vi "Measurement Logic.vi"() -> ()   [LabVIEW 2021, in "niScope EX Getting Started.lvlib"]
uses:
  niScope EX Getting Started.lvlib
  Measurement Configuration.ctl
  Measurement Results.ctl
  <vilib>/Plug-In SDKs/Measurements/Measure Call Context/Measure Call Context.lvclass
  <vilib>/Plug-In SDKs/Sessions/niScope/NI Session Management niScope.lvlib
  <vilib>/Plug-In SDKs/Clients/Session Management V1/Session Reservation/Session Reservation.lvclass
panel:
  out "measure call context out":refnum<class "Measure Call Context.lvclass">
  in  "measure call context in":refnum<class "Measure Call Context.lvclass">
  out "measurement results":T1
  in  "measurement configuration":T2={"Channel(s)"="Lorem ipsum dolor sit", "Simulate?"=TRUE, "resource name Pin"=""}
  out "error out":errorcluster
  in  "error in":errorcluster
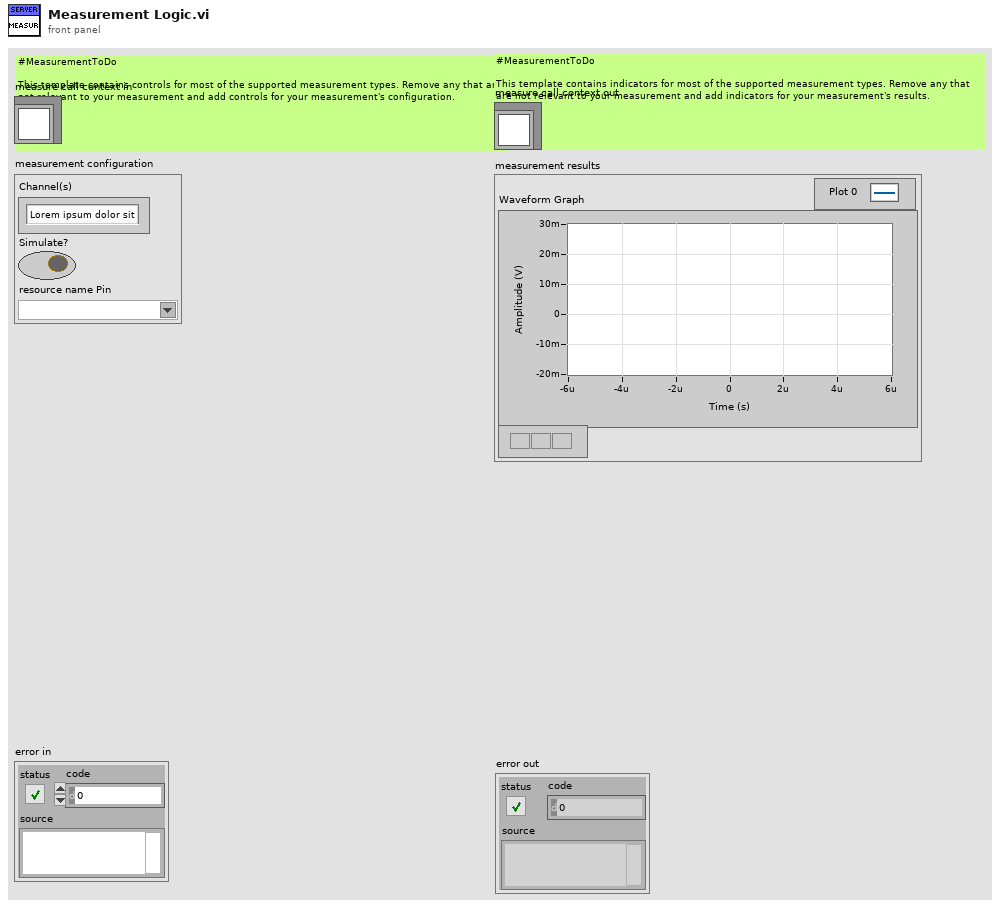
[diagram p1: front panel]
types:
  T1 = typedef "niScope EX Getting Started.lvlib/Measurement Results.ctl" = cluster{"Waveform Graph":cluster{"relativeInitialX":dbl, "xIncrement":dbl, "wfm":dbl[]}[]}
  T2 = typedef "niScope EX Getting Started.lvlib/Measurement Configuration.ctl" = cluster{"Channel(s)":string, "Simulate?":bool, "resource name Pin":string}
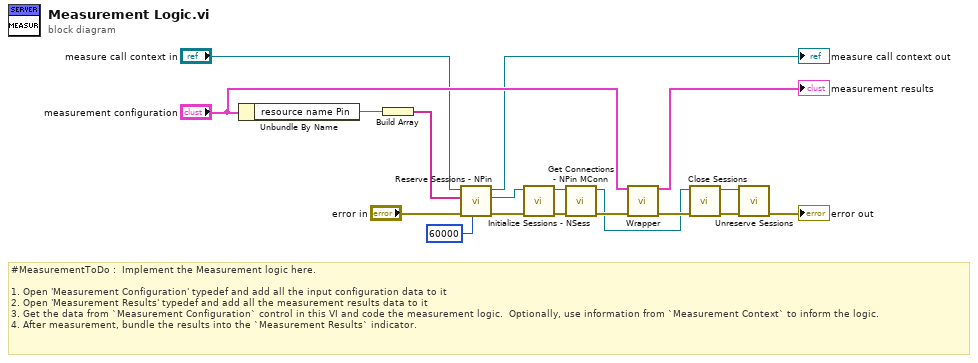
[diagram p0: block diagram]
diagram:
  # "#MeasurementToDo :  Implement the Measurement logic here.\n\n1. Open 'Measurement Configuration' typedef and add all the input configuration data to it\n2. Open 'Measurement Results' typedef and add all the measurement results data to it\n3. Get the data from `Measurement Configuration` control in this VI and code the measurement logic.  Optionally, use information from `Measurement Context` to inform the logic.\n4. After measurement, bundle the results into the `Measurement Results` indicator."
  n1 = Unbundle By Name("measurement configuration") -> ("resource name Pin"=w17:string)
  n2 = Build Array(w17) -> (w14:string[])
  n3 = call <vilib>:"Reserve Sessions - NPin.vi"("timeout (ms)"=60000, "error in"="error in", "pin or relay names"=w14, "measurement context in"="measure call context in") -> ("error out"=w12:errorcluster, "session reservation out"=w2:refnum<class "Session Reservation.lvclass">, "measurement context out"=→"measure call context out":refnum<class "Measure Call Context.lvclass">)  [unwired: 5 in]
  n4 = call <vilib>:"Initialize Sessions - NSess.vi"("error in"=w12, "session reservation in"=w2) -> ("error out"=w11:errorcluster, "session reservation out"=w10:refnum<class "Session Reservation.lvclass">)  [unwired: 6 in, 2 out]
  n5 = call <vilib>:"Get Connections - NPin MConn.vi"("error in"=w11, "session reservation in"=w10) -> ("error out"=w9:errorcluster, "session reservation out"=w3:refnum<class "Session Reservation.lvclass">)  [unwired: 7 in, 1 out]
  n6 = call "Wrapper.vi"("measurement configuration"="measurement configuration", "error in"=w9) -> ("measurement results"=→"measurement results":T1, "error out"=w8:errorcluster)  [unwired: 12 in]
  n7 = call <vilib>:"Close Sessions.vi"("error in"=w8, "session reservation in"=w3) -> ("error out"=w6:errorcluster, "session reservation out"=w5:refnum<class "Session Reservation.lvclass">)  [unwired: 8 in]
  n8 = call <vilib>:"Unreserve Sessions.vi"("error in"=w6, "session reservation in"=w5) -> ("error out"=→"error out":errorcluster)  [unwired: 9 in]
